vi "Delete_From_Array_1D.vi"(9 "Delete from Array 1D":i8[](array[numeric])=[0, 1, 2, 3, 4], 10 "Length":i32, 11 "Index Delete":i32) -> (1 "Deleted Portion 1D":i8[](array[numeric]), 2 "New Array 1D":i8[](array[numeric]))   [LabVIEW 2018]
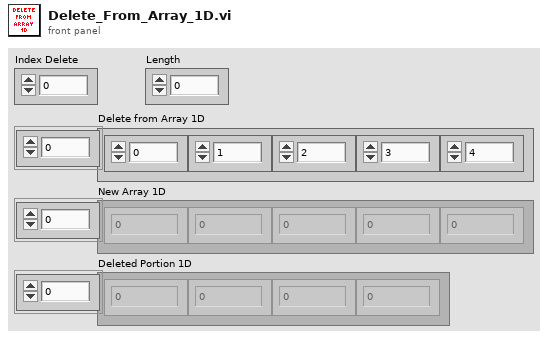
[diagram p1: front panel]
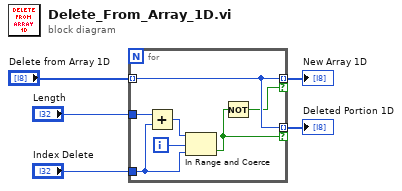
[diagram p0: block diagram]
diagram:
  n1 = for {
    tunnel: "Index Delete" -> [w9]
    tunnel: "Length" -> [w10]
    tunnel: "Delete from Array 1D" -> [w8] mode=indexing
    tunnel: [w8] -> w5 mode=indexing if=w7
    tunnel: [w8] -> w1 mode=indexing if=w6
    i -> [w12]
    n2 = Add(x=w10, y=w9) -> (x+y=w11:i32)
    n3 = In Range and Coerce(upper limit=w11, x=w12, lower limit=w9) -> (In Range?=w6:bool)  [unwired: 1 out]
    n4 = Not(x=w6) -> (.not. x?=w7:bool)
  }
  "New Array 1D" <- w5
  "Deleted Portion 1D" <- w1
